vi "Vision Testing.vi"() -> ()   [LabVIEW 2013]
uses:
  <vilib>/vision/Image Controls.llb/IMAQ Image.ctl
  Documents/UberBots/2012/Code/Final Code/fg_typedef.ctl
  <vilib>/vision/NI_Vision_Development_Module.lvlib
panel:
  out "Image Dst Out":T1(plugin-control)
  out "Image Out 3":T1(plugin-control)
  in  "File Path":path
  out "Sorted Data":dbl[][](array[numeric])
  out "Number of Particles Found":i32
  out "error out 2":errorcluster
  out "Image Out 2":T1(plugin-control)
  out "Number of Hoops Found":i32
  out "error out":errorcluster
  out "Image Out":T1
  in  "error in (no error)":errorcluster
  # "COM X"
  # "COM Y"
types:
  T1 = typedef "IMAQ Image.ctl" = refnum<image>
  T2 = typedef "Image Type" = u32
  T3 = typedef "fg_typedef.ctl" = enum16{"Get", "Set"}
  T4 = enum32{"AutoM", "Close", "Dilate", "Erode", "Gradient", "Gradient out", "Gradient in", "Hit miss", "Open", "PClose", "POpen", "Thick", "Thin"}
  T5 = cluster{"Brightness":sgl, "Contrast":sgl, "Gamma":sgl}
  T6 = cluster{"Measurement Parameter":i32, "Range Lower Value":dbl, "Range Upper Value":dbl, "Range":bool, "Measurement Type":bool}[]
  T7 = typedef "Particle Parameters" = i32
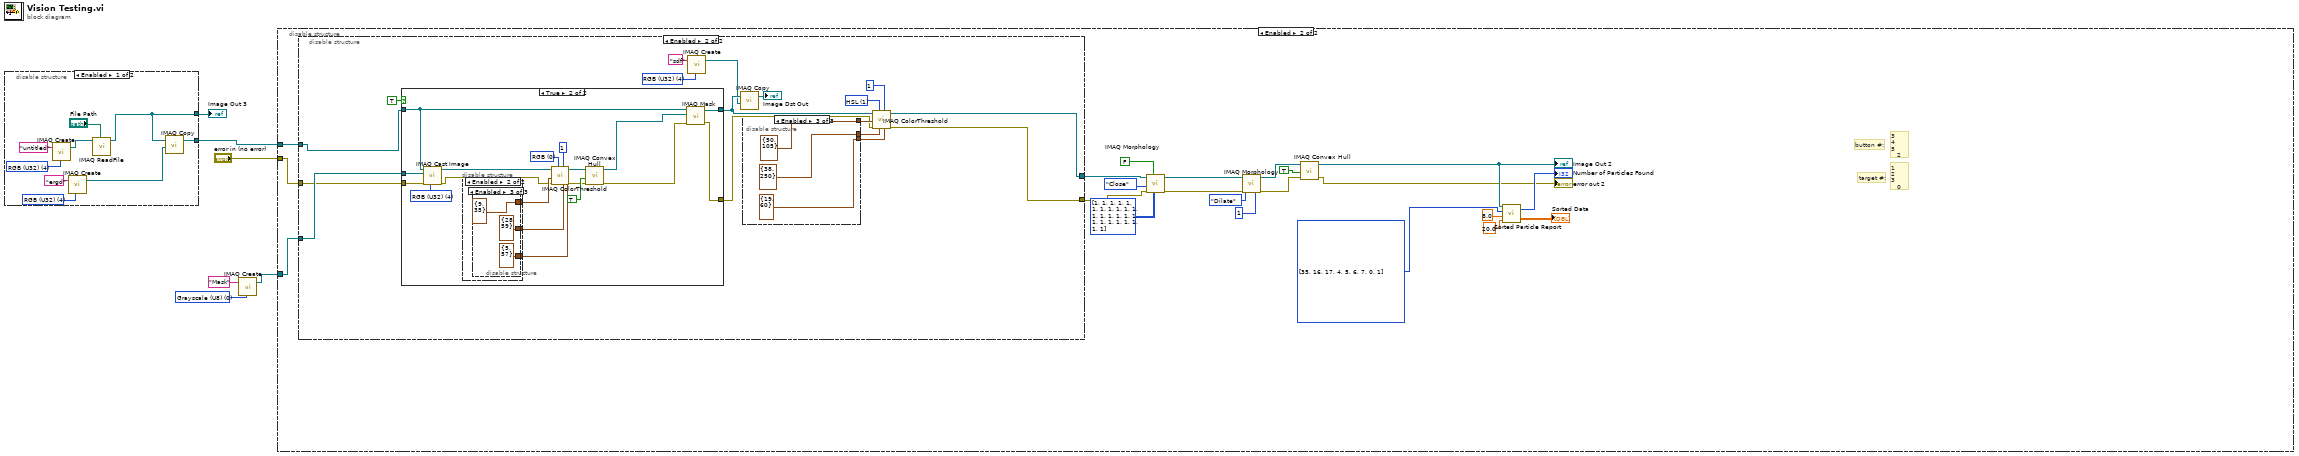
[diagram p0: block diagram]
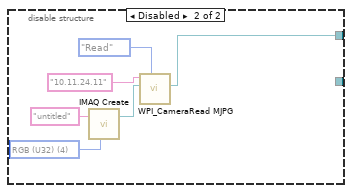
[diagram p2: hidden frame]
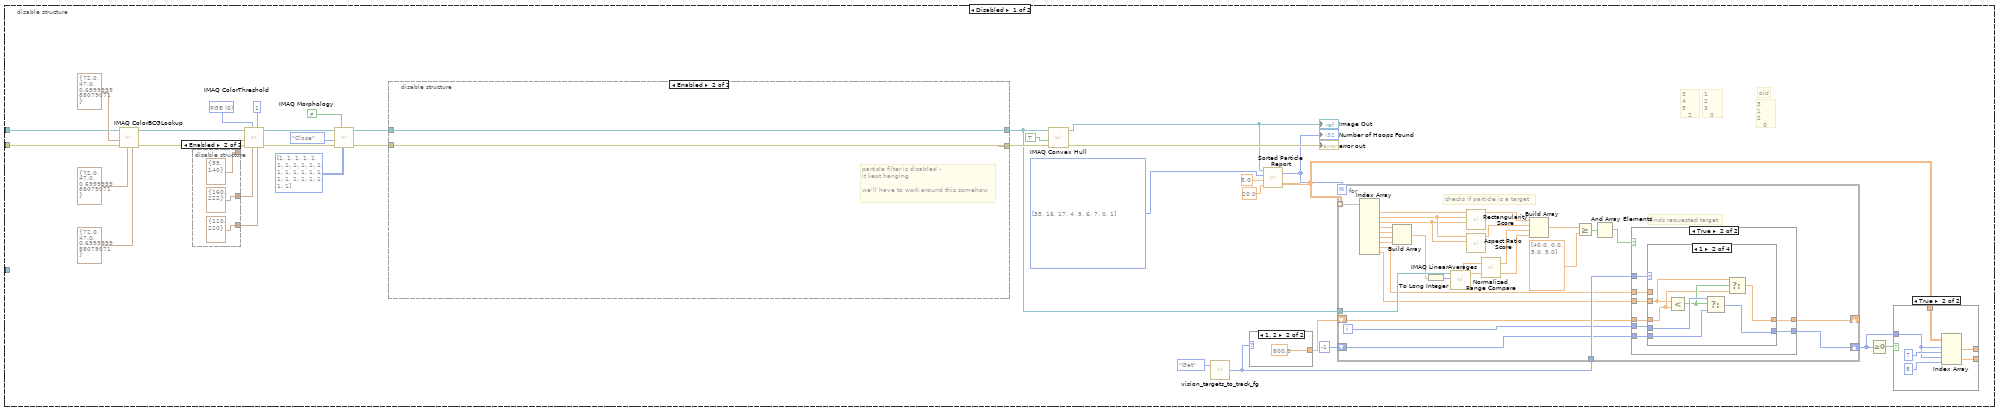
[diagram p3: hidden frame]
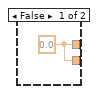
[diagram p4: hidden frame]
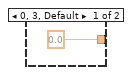
[diagram p5: hidden frame]
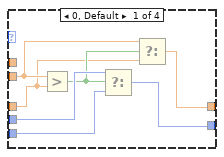
[diagram p7: hidden frame]
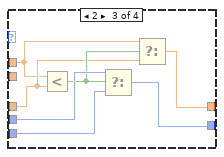
[diagram p8: hidden frame]
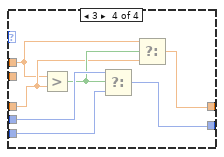
[diagram p9: hidden frame]
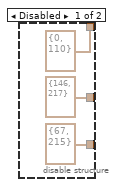
[diagram p10: hidden frame]
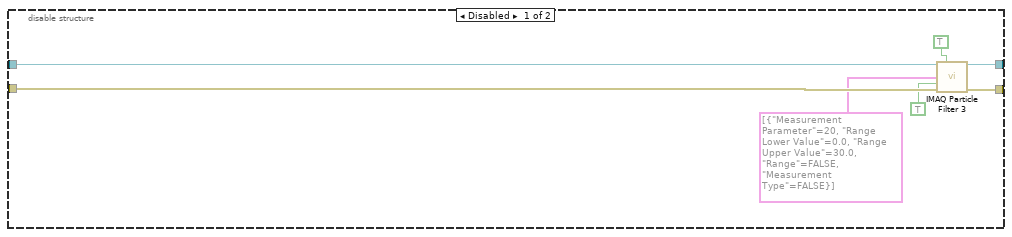
[diagram p11: hidden frame]
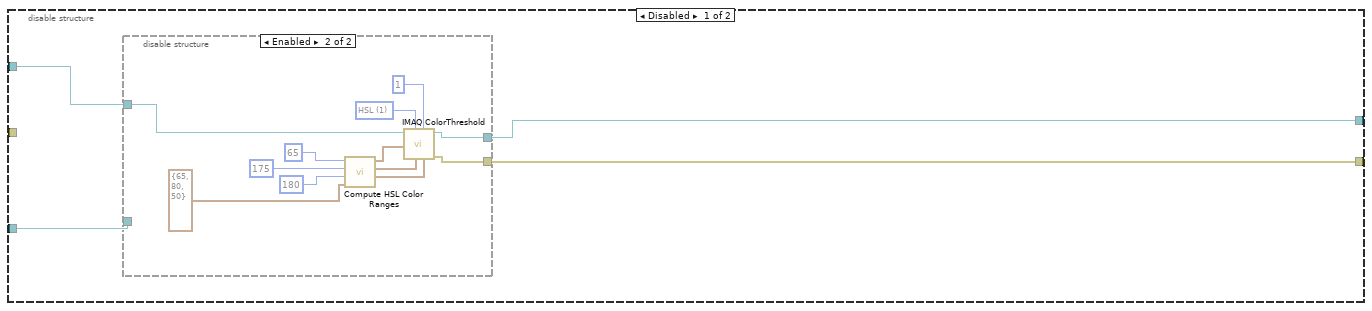
[diagram p12: hidden frame]
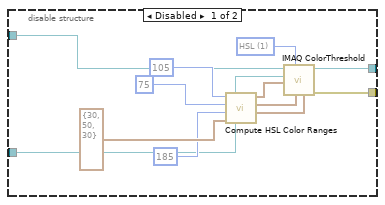
[diagram p13: hidden frame]
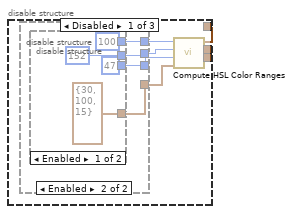
[diagram p14: hidden frame]
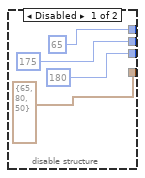
[diagram p15: hidden frame]
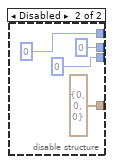
[diagram p16: hidden frame]
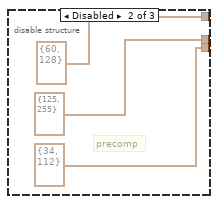
[diagram p17: hidden frame]
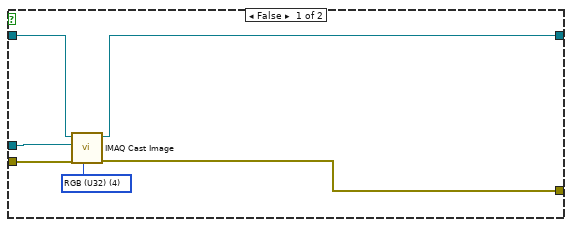
[diagram p18: hidden frame]
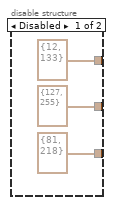
[diagram p19: hidden frame]
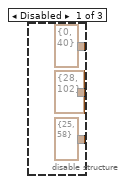
[diagram p20: hidden frame]
diagram:
  w4 = T2 0 items=["Grayscale (U8)", "Grayscale (I16)", "Grayscale (SGL)", "Complex (CSG)", "RGB (U32)", "HSL (U32)", "RGB (U64)", "Grayscale (U16)"] ("Image Type")
  n1 = disable-structure shown="Enabled" {
    disable-tunnel: [w7 _] -> w2
    disable-tunnel: [w11 w16] -> w1
    frame Enabled {
      w9 = T2 4 items=["Grayscale (U8)", "Grayscale (I16)", "Grayscale (SGL)", "Complex (CSG)", "RGB (U32)", "HSL (U32)", "RGB (U64)", "Grayscale (U16)"] ("Image Type")
      w14 = T2 4 items=["Grayscale (U8)", "Grayscale (I16)", "Grayscale (SGL)", "Complex (CSG)", "RGB (U32)", "HSL (U32)", "RGB (U64)", "Grayscale (U16)"] ("Image Type")
      n2 = call "IMAQ Create"("Image Name"="untitled", "Image Type"=w14) -> ("New Image"=w15:T1)  [unwired: 3 in, 1 out]
      n3 = call "IMAQ Create"("Image Name"="ergd", "Image Type"=w9) -> ("New Image"=w8:T1)  [unwired: 3 in, 1 out]
      n4 = call "IMAQ ReadFile"("File Path"="File Path", "Image"=w15) -> ("Image Out"=w11:T1)  [unwired: 5 in, 4 out]
      n5 = call "IMAQ Copy"("Image Dst"=w8, "Image Src"=w11) -> ("Image Dst Out"=w7:T1)  [unwired: 4 in, 1 out]
    }
    frame Disabled {
      w18 = T2 4 items=["Grayscale (U8)", "Grayscale (I16)", "Grayscale (SGL)", "Complex (CSG)", "RGB (U32)", "HSL (U32)", "RGB (U64)", "Grayscale (U16)"] ("Image Type")
      n6 = call "IMAQ Create"("Image Name"="untitled", "Image Type"=w18) -> ("New Image"=w17:T1)  [unwired: 3 in, 1 out]
      n7 = call <vilib>:"WPI_CameraRead MJPG.vi"("Operation"=enum16{"Read", "Reopen", "Close"}."Read", "Image"=w17, "address"="10.11.24.11") -> ("Image Out"=w16:T1)  [unwired: 6 in, 2 out]
    }
  }
  "Image Out 3" <- w1
  n8 = call "IMAQ Create"("Image Name"="Mask", "Image Type"=w4) -> ("New Image"=w3:T1)  [unwired: 2 in, 2 out]
  n9 = disable-structure shown="Enabled" {
    disable-tunnel: "error in (no error)" -> [w39 w151]
    disable-tunnel: w2 -> [w38 w162]
    disable-tunnel: w3 -> [_ w152]
    frame Disabled {
      w31 = T7[] [35, 16, 17, 4, 5, 6, 7, 0, 1] items=["Center of Mass X", "Center of Mass Y", "First Pixel X", "First Pixel Y", "Bounding Rect Left", "Bounding Rect Top", "Bounding Rect Right", "Bounding Rect Bottom", "Max Feret Diameter Start X", "Max Feret Diameter Start Y", "Max Feret Diameter End X", "Max Feret Diameter End Y", "Max Horiz. Segment Length Left", "Max Horiz. Segment Length Right", "Max Horiz. Segment Length Row", "-", "Bounding Rect Width", "Bounding Rect Height", "Bounding Rect Diagonal", "Perimeter", "Convex Hull Perimeter", "Holes' Perimeter", "Max Feret Diameter", "Equivalent Ellipse Major Axis", "Equivalent Ellipse Minor Axis", "Equivalent Ellipse Minor Axis (Feret)", "Equivalent Rect Long Side", "Equivalent Rect Short Side", "Equivalent Rect Diagonal", "Equivalent Rect Short Side (Feret)", "Average Horiz. Segment Length", "Average Vert. Segment Length", "Hydraulic Radius", "Waddel Disk Diameter", "-", "Area", "Holes' Area", "Particle & Holes' Area", "Convex Hull Area", "Image Area", "-", "Number of Holes", "Number of Horiz. Segments", "Number of Vert. Segments", "-", "Orientation", "Max Feret Diameter Orientation", "-", "% Area/Image Area", "% Area/(Particle & Holes' Area)", "Ratio of Equivalent Ellipse Axes", "Ratio of Equivalent Rect Sides", "-", "Elongation Factor", "Compactness Factor", "Heywood Circularity Factor", "Type Factor", "-", "Sum X", "Sum Y", "Sum XX", "Sum XY", "Sum YY", "Sum XXX", "Sum XXY", "Sum XYY", "Sum YYY", "-", "Moment of Inertia XX", "Moment of Inertia XY", "Moment of Inertia YY", "Moment of Inertia XXX", "Moment of Inertia XXY", "Moment of Inertia XYY", "Moment of Inertia YYY", "Norm. Moment of Inertia XX", "Norm. Moment of Inertia XY", "Norm. Moment of Inertia YY", "Norm. Moment of Inertia XXX", "Norm. Moment of Inertia XXY", "Norm. Moment of Inertia XYY", "Norm. Moment of Inertia YYY", "Hu Moment 1", "Hu Moment 2", "Hu Moment 3", "Hu Moment 4", "Hu Moment 5", "Hu Moment 6", "Hu Moment 7"] ("Requested Particle Measurements")
      w53 = u16 0 items=["RGB", "HSL", "HSV", "HSI"] ("Color Mode")
      # "old"
      # "1   \n2     3\n   0"
      # "3   \n1     2\n   0"
      # "3   \n4     5\n   2"
      n10 = call "IMAQ ColorBCGLookup"("Blue BCG Values"=T5 {"Brightness"=72.0, "Contrast"=47.0, "Gamma"=0.7}, "Green BCG Values"=T5 {"Brightness"=72.0, "Contrast"=47.0, "Gamma"=0.7}, "error in (no error)"=w39, "Red BCG Values"=T5 {"Brightness"=72.0, "Contrast"=47.0, "Gamma"=0.7}, "Image Src"=w38) -> ("error out"=w58:errorcluster, "Image Dst Out"=w49:T1)  [unwired: 2 in, 3 out]
      n11 = disable-structure shown="Enabled" {
        disable-tunnel: [cluster{"Lower value":i32, "Upper value":i32} {"Lower value"=0, "Upper value"=110} ("Red or Hue Range") cluster{"Lower value":i32, "Upper value":i32} {"Lower value"=95, "Upper value"=140} ("Red or Hue Range")] -> w52
        disable-tunnel: [cluster{"Lower value":i32, "Upper value":i32} {"Lower value"=146, "Upper value"=217} ("Green or Sat Range") cluster{"Lower value":i32, "Upper value":i32} {"Lower value"=160, "Upper value"=222} ("Green or Sat Range")] -> w51
        disable-tunnel: [cluster{"Lower value":i32, "Upper value":i32} {"Lower value"=67, "Upper value"=215} ("Blue or Luma or Val or Inten Range") cluster{"Lower value":i32, "Upper value":i32} {"Lower value"=110, "Upper value"=220} ("Blue or Luma or Val or Inten Range")] -> w50
        frame Disabled {
        }
        frame Enabled {
        }
      }
      n12 = call "IMAQ ColorThreshold"("Blue or Luma or Val or Inten Range"=w50, "Replace Value"=1, "Green or Sat Range"=w51, "Color Mode"=w53, "error in (no error)"=w58, "Red or Hue Range"=w52, "Image Src"=w49) -> ("error out"=w48:errorcluster, "Image Dst Out"=w44:T1)  [unwired: 1 in, 2 out]
      n13 = call "IMAQ Morphology"("Structuring Element"=i32[][] [[1, 1, 1, 1, 1], [1, 1, 1, 1, 1], [1, 1, 1, 1, 1], [1, 1, 1, 1, 1], [1, 1, 1, 1, 1]], "Square/Hexa (Square)"=FALSE, "error in (no error)"=w48, "Operation"=T4."Close", "Image Src"=w44) -> ("error out"=w43:errorcluster, "Image Dst Out"=w41:T1)  [unwired: 2 in, 3 out]
      n14 = disable-structure shown="Enabled" {
        disable-tunnel: w43 -> [w147 w149]
        disable-tunnel: [w144 w149] -> w42
        disable-tunnel: w41 -> [w143 w148]
        disable-tunnel: [w141 w148] -> w37
        frame Disabled {
          n15 = call "IMAQ Particle Filter 3"("Image Src"=w143, "Connectivity 4/8 (8)"=TRUE, "Selection Values"=T6 [{"Measurement Parameter"=20, "Range Lower Value"=0.0, "Range Upper Value"=30.0, "Range"=FALSE, "Measurement Type"=FALSE}], "Keep/Remove Particles (F)"=TRUE ("Keep/Remove Particles"), "error in (no error)"=w147) -> ("Image Dst Out"=w141:T1, "error out"=w144:errorcluster)  [unwired: 4 in, 5 out]
        }
        frame Enabled {
          # "particle filter is disabled - \nit kept hanging\n\nwe'll have to work around this somehow"
        }
      }
      n16 = call "IMAQ Convex Hull"("error in (no error)"=w42, "Connectivity 4/8 (8)"=TRUE, "Image Src"=w37) -> ("error out"=→"error out":errorcluster, "Image Dst Out"=w22:T1)  [unwired: 1 in, 6 out]
      "Image Out" <- w22
      n17 = call "vision_targets_to_track_fg.vi"("Menu (Get)"=fg_typedef."Get") -> ("Output"=w34:i32)  [unwired: 1 in]
      n18 = case shown="1, 2" w34 {
        tunnel: [0.0 ("element") 800.0 ("element")] -> w35
        frame 0, 3, Default {
        }
        frame 1, 2 {
        }
      }
      n19 = call "Sorted Particle Report.vi"("Area Size Limit"=20.0, "Particle Count Limit"=8.0, "Pixel Measurements"=w31, "Image in"=w22) -> ("Sorted Data"=w27:dbl[][], "Particles"=w28:i32)
      "Number of Hoops Found" <- w28
      n20 = for {
        N: w28 -> [_]
        tunnel: w37 -> [w96]
        tunnel: w27 -> [w95] mode=indexing
        tunnel: w34 -> [w85]
        shift-right: [w77] -> _
        shift-left: w35 -> [w80]
        shift-right: [w78] -> w26
        shift-left: -1 -> [w79]
        i -> [w81]
        # "checks if particle is a target"
        # "finds requested target"
        n21 = Index Array(array=w95) -> (element #1=w76:dbl, element #2=w73:dbl, element #3=w72:dbl, element #4=w91:dbl, element #5=w90:dbl, element #6=w89:dbl, element #7=w88:dbl, element #8=w83:dbl, element #9=w84:dbl)  [unwired: 9 in]
        n22 = Build Array(w91, w90, w89, w88) -> (w87:dbl[])
        n23 = To Long Integer(number=w87) -> (32bit integer=w86:i32[])
        n24 = call "IMAQ LinearAverages"("Optional Rectangle"=w86, "Image Src"=w96) -> ("Y Axis Averages"=w68:sgl[], "X Axis Averages"=w69:sgl[])  [unwired: 2 in, 6 out]
        n25 = call "Rectangularity Score.vi"("Height"=w72, "Width"=w73, "Area"=w76) -> ("Score"=w75:dbl)  [unwired: 8 in]
        n26 = call "Aspect Ratio Score.vi"("Height"=w72, "Width"=w73) -> ("Score"=w74:dbl)  [unwired: 9 in]
        n27 = call "Normalized Range Compare.vi"("Y Averages"=w68, "X Averages"=w69) -> ("Y Score"=w70:dbl, "X Score"=w71:dbl)
        n28 = Build Array(w75, w74, w71, w70) -> (w94:dbl[])
        n29 = Greater Or Equal?(x=w94, y=dbl[] [40.0, 0.0, 5.0, 5.0]) -> (x >= y?=w92:bool[])
        n30 = And Array Elements(Boolean array=w92) -> (logical AND=w82:bool)
        n31 = case shown="True" w82 {
          tunnel: w85 -> [_ w106]
          tunnel: w84 -> [_ w105]
          tunnel: w83 -> [_ w104]
          tunnel: w81 -> [_ w103]
          tunnel: w80 -> [w97 w102]
          tunnel: w79 -> [w98 w101]
          tunnel: [w98 w100] -> w78
          tunnel: [w97 w99] -> w77
          frame False {
          }
          frame True {
            n32 = case shown="1" w106 {
              tunnel: w105 -> [w109 w114 _ _]
              tunnel: w104 -> [_ _ w121 w128]
              tunnel: w103 -> [w113 w120 w127 w134]
              tunnel: w102 -> [w108 w116 w123 w130]
              tunnel: w101 -> [w112 w119 w126 w133]
              tunnel: [w111 w118 w125 w132] -> w100
              tunnel: [w107 w115 w122 w129] -> w99
              frame 0, Default {
                n33 = Greater?(x=w109, y=w108) -> (0:w110:bool)
                n34 = Select(t=w113, s=w110, f=w112) -> (s? t:f=w111:i32)
                n35 = Select(t=w109, s=w110, f=w108) -> (s? t:f=w107:dbl)
              }
              frame 1 {
                n36 = Less?(x=w114, y=w116) -> (x < y?=w117:bool)
                n37 = Select(t=w120, s=w117, f=w119) -> (s? t:f=w118:i32)
                n38 = Select(t=w114, s=w117, f=w116) -> (s? t:f=w115:dbl)
              }
              frame 2 {
                n39 = Less?(x=w121, y=w123) -> (x < y?=w124:bool)
                n40 = Select(t=w127, s=w124, f=w126) -> (s? t:f=w125:i32)
                n41 = Select(t=w121, s=w124, f=w123) -> (s? t:f=w122:dbl)
              }
              frame 3 {
                n42 = Greater?(x=w128, y=w130) -> (0:w131:bool)
                n43 = Select(t=w134, s=w131, f=w133) -> (s? t:f=w132:i32)
                n44 = Select(t=w128, s=w131, f=w130) -> (s? t:f=w129:dbl)
              }
            }
          }
        }
      }
      n45 = Greater Or Equal To 0?(x=w26) -> (x >= 0?=w25:bool)
      n46 = case shown="True" w25 {
        tunnel: [w59 w63] -> w24
        tunnel: [w59 w62] -> w23
        tunnel: w27 -> [_ w61]
        tunnel: w26 -> [_ w60]
        frame False {
          w59 = 0.0 ("Numeric")
        }
        frame True {
          n47 = Index Array(array=w61, index (row) #1=w60, index (col) #1=7, index (row) #2=w60, index (col) #2=8) -> (element #1=w63:dbl, element #2=w62:dbl)
        }
      }
    }
    frame Enabled {
      w161 = T7[] [35, 16, 17, 4, 5, 6, 7, 0, 1] items=["Center of Mass X", "Center of Mass Y", "First Pixel X", "First Pixel Y", "Bounding Rect Left", "Bounding Rect Top", "Bounding Rect Right", "Bounding Rect Bottom", "Max Feret Diameter Start X", "Max Feret Diameter Start Y", "Max Feret Diameter End X", "Max Feret Diameter End Y", "Max Horiz. Segment Length Left", "Max Horiz. Segment Length Right", "Max Horiz. Segment Length Row", "-", "Bounding Rect Width", "Bounding Rect Height", "Bounding Rect Diagonal", "Perimeter", "Convex Hull Perimeter", "Holes' Perimeter", "Max Feret Diameter", "Equivalent Ellipse Major Axis", "Equivalent Ellipse Minor Axis", "Equivalent Ellipse Minor Axis (Feret)", "Equivalent Rect Long Side", "Equivalent Rect Short Side", "Equivalent Rect Diagonal", "Equivalent Rect Short Side (Feret)", "Average Horiz. Segment Length", "Average Vert. Segment Length", "Hydraulic Radius", "Waddel Disk Diameter", "-", "Area", "Holes' Area", "Particle & Holes' Area", "Convex Hull Area", "Image Area", "-", "Number of Holes", "Number of Horiz. Segments", "Number of Vert. Segments", "-", "Orientation", "Max Feret Diameter Orientation", "-", "% Area/Image Area", "% Area/(Particle & Holes' Area)", "Ratio of Equivalent Ellipse Axes", "Ratio of Equivalent Rect Sides", "-", "Elongation Factor", "Compactness Factor", "Heywood Circularity Factor", "Type Factor", "-", "Sum X", "Sum Y", "Sum XX", "Sum XY", "Sum YY", "Sum XXX", "Sum XXY", "Sum XYY", "Sum YYY", "-", "Moment of Inertia XX", "Moment of Inertia XY", "Moment of Inertia YY", "Moment of Inertia XXX", "Moment of Inertia XXY", "Moment of Inertia XYY", "Moment of Inertia YYY", "Norm. Moment of Inertia XX", "Norm. Moment of Inertia XY", "Norm. Moment of Inertia YY", "Norm. Moment of Inertia XXX", "Norm. Moment of Inertia XXY", "Norm. Moment of Inertia XYY", "Norm. Moment of Inertia YYY", "Hu Moment 1", "Hu Moment 2", "Hu Moment 3", "Hu Moment 4", "Hu Moment 5", "Hu Moment 6", "Hu Moment 7"] ("Requested Particle Measurements")
      # "target #:"
      # "button #:"
      # "1   \n2     3\n   0"
      # "3   \n4     5\n   2"
      n48 = disable-structure shown="Enabled" {
        disable-tunnel: [w175 w207] -> w168
        disable-tunnel: [w174 w208] -> w167
        disable-tunnel: w162 -> [w173 w205]
        disable-tunnel: w152 -> [w172 w216]
        disable-tunnel: w151 -> [_ w215]
        frame Disabled {
          n49 = disable-structure shown="Enabled" {
            disable-tunnel: [w187 w190] -> w175
            disable-tunnel: [w186 w191] -> w174
            disable-tunnel: w173 -> [w177 w189]
            disable-tunnel: w172 -> [w176 _]
            frame Disabled {
              w185 = u16 1 items=["RGB", "HSL", "HSV", "HSI"] ("Color Mode")
              n50 = call "Compute HSL Color Ranges.vi"("Margins"=cluster{"Hue":i32, "Sat":i32, "Lum":i32} {"Hue"=30, "Sat"=50, "Lum"=30}, "Luminance"=185, "Saturation"=75, "Hue"=105) -> ("Lum Range"=w182:cluster{i32, i32}, "Sat Range"=w183:cluster{i32, i32}, "Hue Range"=w184:cluster{i32, i32})  [unwired: 5 in]
              n51 = call "IMAQ ColorThreshold"("Blue or Luma or Val or Inten Range"=w182, "Green or Sat Range"=w183, "Color Mode"=w185, "Red or Hue Range"=w184, "Image Dst"=w176, "Image Src"=w177) -> ("error out"=w187:errorcluster, "Image Dst Out"=w186:T1)  [unwired: 4 in]
            }
            frame Enabled {
              w193 = u16 1 items=["RGB", "HSL", "HSV", "HSI"] ("Color Mode")
              n52 = call "Compute HSL Color Ranges.vi"("Margins"=cluster{"Hue":i32, "Sat":i32, "Lum":i32} {"Hue"=65, "Sat"=80, "Lum"=50}, "Luminance"=180, "Saturation"=175, "Hue"=65) -> ("Lum Range"=w196:cluster{i32, i32}, "Sat Range"=w195:cluster{i32, i32}, "Hue Range"=w194:cluster{i32, i32})  [unwired: 5 in]
              n53 = call "IMAQ ColorThreshold"("Blue or Luma or Val or Inten Range"=w196, "Replace Value"=1, "Green or Sat Range"=w195, "Color Mode"=w193, "Red or Hue Range"=w194, "Image Src"=w189) -> ("error out"=w190:errorcluster, "Image Dst Out"=w191:T1)  [unwired: 4 in]
            }
          }
        }
        frame Enabled {
          w203 = T2 4 items=["Grayscale (U8)", "Grayscale (I16)", "Grayscale (SGL)", "Complex (CSG)", "RGB (U32)", "HSL (U32)", "RGB (U64)", "Grayscale (U16)"] ("Image Type")
          w211 = u16 1 items=["RGB", "HSL", "HSV", "HSI"] ("Color Mode")
          n54 = case shown="True" TRUE {
            tunnel: [w248 w269] -> w204
            tunnel: w216 -> [w250 w261]
            tunnel: w205 -> [w249 w260]
            tunnel: [w247 w256] -> w209
            tunnel: w215 -> [w246 w253]
            frame False {
              w251 = T2 4 items=["Grayscale (U8)", "Grayscale (I16)", "Grayscale (SGL)", "Complex (CSG)", "RGB (U32)", "HSL (U32)", "RGB (U64)"] ("Image Type")
              n55 = call "IMAQ Cast Image"("Image Type"=w251, "error in (no error)"=w246, "Image Dst"=w250, "Image Src"=w249) -> ("error out"=w247:errorcluster, "Image Dst Out"=w248:T1)  [unwired: 6 in]
            }
            frame True {
              w266 = u16 0 items=["RGB", "HSL", "HSV", "HSI"] ("Color Mode")
              w268 = T2 4 items=["Grayscale (U8)", "Grayscale (I16)", "Grayscale (SGL)", "Complex (CSG)", "RGB (U32)", "HSL (U32)", "RGB (U64)"] ("Image Type")
              n56 = call "IMAQ Cast Image"("Image Type"=w268, "error in (no error)"=w253, "Image Dst"=w261, "Image Src"=w260) -> ("error out"=w254:errorcluster, "Image Dst Out"=w264:T1)  [unwired: 6 in]
              n57 = disable-structure shown="Enabled" {
                disable-tunnel: [cluster{"Lower value":i32, "Upper value":i32} {"Lower value"=12, "Upper value"=133} ("Red or Hue Range") w275] -> w258
                disable-tunnel: [cluster{"Lower value":i32, "Upper value":i32} {"Lower value"=127, "Upper value"=255} ("Green or Sat Range") w274] -> w257
                disable-tunnel: [cluster{"Lower value":i32, "Upper value":i32} {"Lower value"=81, "Upper value"=218} ("Blue or Luma or Val or Inten Range") w273] -> w252
                frame Disabled {
                }
                frame Enabled {
                  n58 = disable-structure shown="Enabled" {
                    disable-tunnel: [cluster{"Lower value":i32, "Upper value":i32} {"Lower value"=0, "Upper value"=40} ("Red or Hue Range") cluster{"Lower value":i32, "Upper value":i32} {"Lower value"=0, "Upper value"=68} ("Red or Hue Range") cluster{"Lower value":i32, "Upper value":i32} {"Lower value"=9, "Upper value"=35} ("Red or Hue Range")] -> w275
                    disable-tunnel: [cluster{"Lower value":i32, "Upper value":i32} {"Lower value"=28, "Upper value"=102} ("Green or Sat Range") cluster{"Lower value":i32, "Upper value":i32} {"Lower value"=62, "Upper value"=195} ("Green or Sat Range") cluster{"Lower value":i32, "Upper value":i32} {"Lower value"=28, "Upper value"=59} ("Green or Sat Range")] -> w274
                    disable-tunnel: [cluster{"Lower value":i32, "Upper value":i32} {"Lower value"=25, "Upper value"=58} ("Blue or Luma or Val or Inten Range") cluster{"Lower value":i32, "Upper value":i32} {"Lower value"=0, "Upper value"=86} ("Blue or Luma or Val or Inten Range") cluster{"Lower value":i32, "Upper value":i32} {"Lower value"=5, "Upper value"=57} ("Blue or Luma or Val or Inten Range")] -> w273
                    frame Disabled {
                    }
                    frame Disabled {
                      # "pre"
                    }
                    frame Enabled {
                    }
                  }
                }
              }
              n59 = call "IMAQ ColorThreshold"("Blue or Luma or Val or Inten Range"=w252, "Replace Value"=1, "Green or Sat Range"=w257, "Color Mode"=w266, "error in (no error)"=w254, "Red or Hue Range"=w258, "Image Src"=w264) -> ("error out"=w262:errorcluster, "Image Dst Out"=w263:T1)  [unwired: 1 in, 2 out]
              n60 = call "IMAQ Convex Hull"("error in (no error)"=w262, "Connectivity 4/8 (8)"=TRUE, "Image Src"=w263) -> ("error out"=w255:errorcluster, "Image Dst Out"=w259:T1)  [unwired: 7 in]
              n61 = call "IMAQ Mask"("error in (no error)"=w255, "Image Mask"=w259, "Image Src"=w260) -> ("error out"=w256:errorcluster, "Image Dst Out"=w269:T1)  [unwired: 2 in]
            }
          }
          n62 = call "IMAQ Create"("Image Name"="sdf", "Image Type"=w203) -> ("New Image"=w201:T1)  [unwired: 3 in, 1 out]
          n63 = call "IMAQ Copy"("Image Dst"=w201, "Image Src"=w204) -> ("Image Dst Out"=→"Image Dst Out":T1)  [unwired: 4 in, 1 out]
          n64 = disable-structure shown="Enabled" {
            disable-tunnel: [w219 cluster{"Lower value":i32, "Upper value":i32} {"Lower value"=34, "Upper value"=112} ("Blue or Luma or Val or Inten Range") cluster{"Lower value":i32, "Upper value":i32} {"Lower value"=19, "Upper value"=60} ("Blue or Luma or Val or Inten Range")] -> w214
            disable-tunnel: [w218 cluster{"Lower value":i32, "Upper value":i32} {"Lower value"=125, "Upper value"=255} ("Green or Sat Range") cluster{"Lower value":i32, "Upper value":i32} {"Lower value"=38, "Upper value"=250} ("Green or Sat Range")] -> w213
            disable-tunnel: [w217 cluster{"Lower value":i32, "Upper value":i32} {"Lower value"=60, "Upper value"=128} ("Red or Hue Range") cluster{"Lower value":i32, "Upper value":i32} {"Lower value"=50, "Upper value"=105} ("Red or Hue Range")] -> w212
            frame Disabled {
              n65 = disable-structure shown="Enabled" {
                disable-tunnel: [65 ("Hue") w231] -> w223
                disable-tunnel: [175 ("Saturation") w230] -> w222
                disable-tunnel: [180 ("Luminance") w229] -> w221
                disable-tunnel: [cluster{"Hue":i32, "Sat":i32, "Lum":i32} {"Hue"=65, "Sat"=80, "Lum"=50} ("Margins") w228] -> w220
                frame Disabled {
                }
                frame Enabled {
                  n66 = disable-structure shown="Enabled" {
                    disable-tunnel: [100 ("Hue") 0 ("Hue")] -> w231
                    disable-tunnel: [152 ("Saturation") 0 ("Saturation")] -> w230
                    disable-tunnel: [47 ("Luminance") 0 ("Luminance")] -> w229
                    disable-tunnel: [cluster{"Hue":i32, "Sat":i32, "Lum":i32} {"Hue"=30, "Sat"=100, "Lum"=15} ("Margins") cluster{"Hue":i32, "Sat":i32, "Lum":i32} {"Hue"=0, "Sat"=0, "Lum"=0} ("Margins")] -> w228
                    frame Enabled {
                    }
                    frame Disabled {
                    }
                  }
                }
              }
              n67 = call "Compute HSL Color Ranges.vi"("Margins"=w220, "Luminance"=w221, "Saturation"=w222, "Hue"=w223) -> ("Lum Range"=w219:cluster{i32, i32}, "Sat Range"=w218:cluster{i32, i32}, "Hue Range"=w217:cluster{i32, i32})  [unwired: 5 in]
            }
            frame Disabled {
              # "precomp"
            }
            frame Enabled {
            }
          }
          n68 = call "IMAQ ColorThreshold"("Blue or Luma or Val or Inten Range"=w214, "Replace Value"=1, "Green or Sat Range"=w213, "Color Mode"=w211, "error in (no error)"=w209, "Red or Hue Range"=w212, "Image Src"=w204) -> ("error out"=w207:errorcluster, "Image Dst Out"=w208:T1)  [unwired: 3 in]
        }
      }
      n69 = call "IMAQ Morphology"("Structuring Element"=i32[][] [[1, 1, 1, 1, 1], [1, 1, 1, 1, 1], [1, 1, 1, 1, 1], [1, 1, 1, 1, 1], [1, 1, 1, 1, 1]], "Square/Hexa (Square)"=FALSE, "error in (no error)"=w168, "Operation"=T4."Close", "Image Src"=w167) -> ("error out"=w155:errorcluster, "Image Dst Out"=w157:T1)  [unwired: 2 in, 3 out]
      n70 = call "IMAQ Morphology"("Number of iterations (1)"=1, "error in (no error)"=w155, "Operation"=T4."Dilate", "Image Src"=w157) -> ("error out"=w154:errorcluster, "Image Dst Out"=w156:T1)  [unwired: 6 in]
      n71 = call "IMAQ Convex Hull"("error in (no error)"=w154, "Connectivity 4/8 (8)"=TRUE, "Image Src"=w156) -> ("error out"=→"error out 2":errorcluster, "Image Dst Out"=w160:T1)  [unwired: 1 in, 6 out]
      "Image Out 2" <- w160
      n72 = call "Sorted Particle Report.vi"("Area Size Limit"=20.0, "Particle Count Limit"=8.0, "Pixel Measurements"=w161, "Image in"=w160) -> ("Sorted Data"=→"Sorted Data":dbl[][], "Particles"=→"Number of Particles Found":i32)
    }
  }
